vi "UTILITY String to Array.vi"(7 "Delimiter":string=" ", 10 "String":string="Time UpperElement LowerElement Compressor Fan1RPM Fan2RPM SetPoint T2(TankSensor) T3A(EvapIn) T3B(EvapOut) T4(CompressorDischarge) T5(Ambient)") -> (2 "Array":string[](array[string]))   [LabVIEW 2016]
uses:
  <vilib>/Utility/error.llb/whitespace.ctl
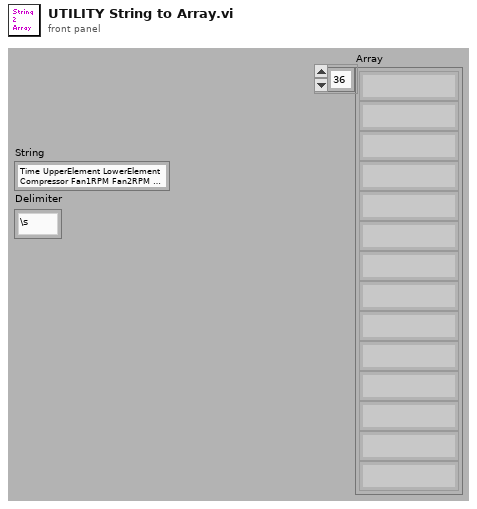
[diagram p1: front panel]
types:
  T1 = typedef "whitespace.ctl" = u16
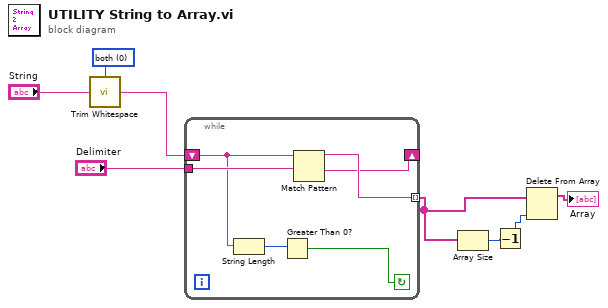
[diagram p0: block diagram]
diagram:
  w5 = T1 0 items=["both", "start of string", "end of string"] ("location (both)")
  n1 = call <vilib>:"Trim Whitespace.vi"("string"="String", "location (both)"=w5) -> ("trimmed string"=w7:string)
  n2 = while {
    tunnel: "Delimiter" -> [w14]
    shift-right: [w9] -> _
    shift-left: w7 -> [w11]
    tunnel: [w13] -> w4 mode=indexing
    stop <- w10 continue-if-true
    n3 = String Length(string=w11) -> (length=w12:i32)
    n4 = Greater Than 0?(x=w12) -> (x > 0?=w10:bool)
    n5 = Match Pattern(string=w11, regular expression=w14) -> (before substring=w13:string, after substring=w9:string)  [unwired: 1 in, 2 out]
  }
  n6 = Array Size(array=w4) -> (size(s)=w2:i32)
  n7 = Decrement(x=w2) -> (x-1=w1:i32)
  n8 = Delete From Array(array=w4, index=w1) -> (array with subset deleted=→"Array":string[])  [unwired: 1 in, 1 out]
